vi "Module Top Level.vi"(8 "error in":errorcluster) -> (0 "error out":errorcluster)   [LabVIEW 2018, in "Testing UI 3.lvlib"]
doc: "This is the top level VI for this module. It uses a queue for communications and is stopped user a user event. The general architecture is similar to a simple queued message handler.\n\nThe VIs associated with this module are organized in a LabVIEW Library."
uses:
  Testing UI 3.lvlib
  Private Controls/UI 3 Data.ctl
  Top Level/Shared Controls/APU Setup File.ctl
  Private Controls/Cutoff Frequency.ctl
  Public Controls/Accel Config.ctl
  Private Controls/Module Data.ctl
  Private Controls/Module Action.ctl
  Globals/Host Globals.vi
  Error Handler/Error Handler.lvlib
  File IO/File IO.lvlib
  UDP Writer/PC UDP Writer.lvlib
panel:
  in  "Channel Select":enum16{"Power Section", "Gearbox", "Fan"}(ring)
  in  "Save Accel Config":bool
  in  "Fan Cutoff Frequency":T1={"LP Passband"=1200.0, "HP Stopband"=250.0, "LP Stopband"=1300.0, "HP Passband"=300.0} {"HP Passband" min=1.0 step=1.0 format="%#.4f"; "LP Stopband" min=1.0 step=1.0 format="%#.4f"; "HP Stopband" min=1.0 step=1.0 format="%#.4f"; "LP Passband" min=1.0 step=1.0 format="%#.4f"}
  in  "GB Cutoff Frequency":T1={"LP Passband"=1200.0, "HP Stopband"=250.0, "LP Stopband"=1300.0, "HP Passband"=300.0} {"HP Passband" min=1.0 step=1.0 format="%#.4f"; "LP Stopband" min=1.0 step=1.0 format="%#.4f"; "HP Stopband" min=1.0 step=1.0 format="%#.4f"; "LP Passband" min=1.0 step=1.0 format="%#.4f"}
  in  "PS Cutoff Frequency":T1={"LP Passband"=1200.0, "HP Stopband"=250.0, "LP Stopband"=1300.0, "HP Passband"=300.0} {"HP Passband" min=1.0 step=1.0 format="%#.4f"; "LP Stopband" min=1.0 step=1.0 format="%#.4f"; "HP Stopband" min=1.0 step=1.0 format="%#.4f"; "LP Passband" min=1.0 step=1.0 format="%#.4f"}
  in  "Units Select":string(combo)="0"
  in  "Show Accel?":bool
  out "Accel Cluster":T2
  in  "FAN Sens":dbl=0.0001 caption="Sensitivity (mV/ms-2)" min=0.0001 format="%#.4f"
  in  "GB Sens":dbl=0.0001 caption="Sensitivity (mV/ms-2)" min=0.0001 format="%#.4f"
  in  "PS Sens":dbl=0.0001 caption="Sensitivity (mV/ms-2)" min=0.0001 format="%#.4f"
  out "UI 3 Data":T3
  out "Fan Peak":dbl caption="Velocity PEAK" format="%.2f"
  out "GB RMS":dbl caption="Velocity RMS" format="%.2f"
  out "PS RMS":dbl caption="Velocity RMS" format="%.2f"
  out "Fan RMS Level":dbl(graph)=0.00041195687684329 caption="peaks"
  out "Gearbox RMS Level":dbl(graph)=0.0759733513075506 caption="peaks"
  out "Power Section RMS Level":dbl(graph)=0.022015968164997 caption="peaks"
  out "Fan Peak":dbl(graph)=0.00138609479700936 caption="peaks"
  out "Gearbox Peak":dbl(graph)=0.40103459883114 caption="peaks"
  out "Power Section Peak":dbl(graph)=0.0689049138645727 caption="peaks"
  out "STOP":bool
  # "Vibration Analysis"
  # "Highpass Cutoff Frequency"
  # "Lowpass Cutoff Frequency"
  # "Highpass Cutoff Frequency"
  # "Lowpass Cutoff Frequency"
  # "Highpass Cutoff Frequency"
  # "Lowpass Cutoff Frequency"
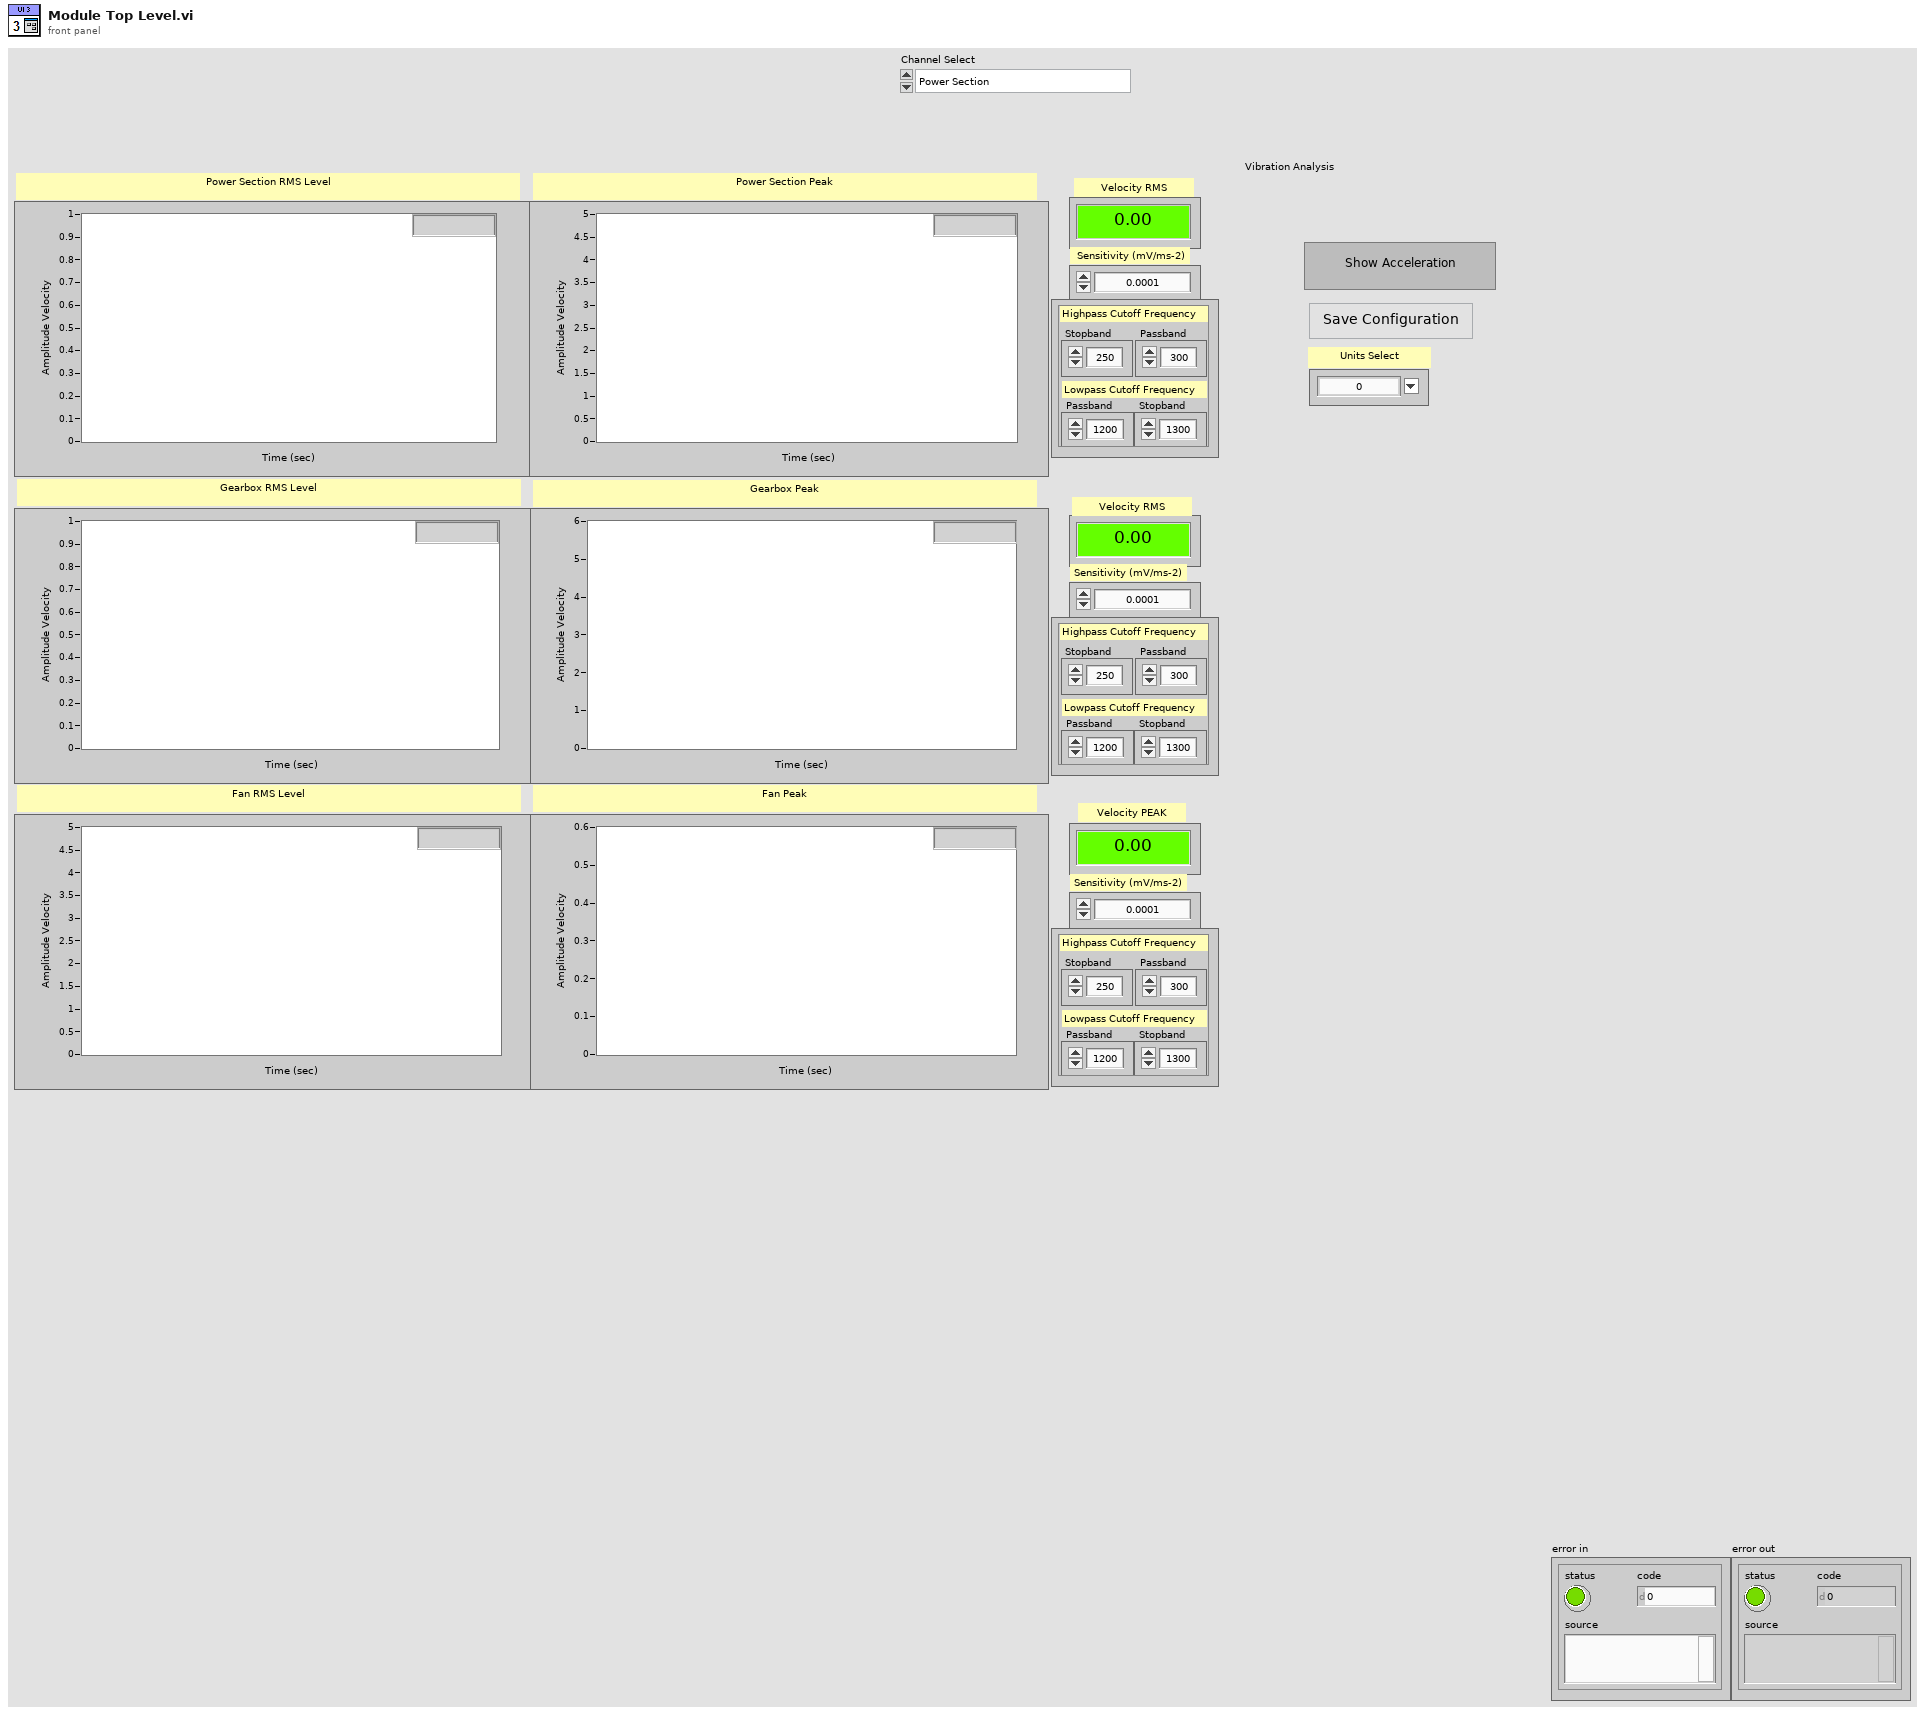
[diagram p1: front panel]
types:
  T1 = typedef "Testing UI 3.lvlib/Cutoff Frequency.ctl" = cluster{"LP Passband":dbl, "HP Stopband":dbl, "LP Stopband":dbl, "HP Passband":dbl}
  T2 = cluster{"Power Section Accel RMS":dbl, "Power Section Accel Peak":dbl, "Gearbox Accel RMS":dbl, "Gearbox Accel Peak":dbl, "Fan Accel RMS":dbl, "Fan Accel Peak":dbl}
  T3 = typedef "Testing UI 3.lvlib/UI 3 Data.ctl" = cluster{"APU Setup File":T4}
  T4 = typedef "APU Setup File.ctl" = cluster{"Sensor Info":string[][], "Variables":string[][], "CMM Table 106":string[][], "CMM Table 106B ":string[][], "Accel Config":string[][], "Report Sheet 1":string[][], "Report Sheet 2":string[][], "Report Sheet 3":string[][]}
  T5 = typedef "Testing UI 3.lvlib/Accel Config.ctl" = cluster{"PS Sens":dbl, "GB Sens":dbl, "FAN Sens":dbl, "PS Cutoff Frequency":T1, "GB Cutoff Frequency":T1, "Fan Cutoff Frequency":T1}
  T6 = enum32{"Invalid", "Standard", "Closed", "Hidden", "Minimized", "Maximized"}
  T7 = typedef "Testing UI 3.lvlib/Module Data.ctl" = cluster{"Data":variant, "Action":T8}
  T8 = typedef "Testing UI 3.lvlib/Module Action.ctl" = enum8{"Init", "Open FP", "Timeout", "Error", "Exit", "Load APU Setup"}
  T9 = typedef "All Data Cluster.ctl" = cluster{"AI":T10, "Accel Data":cluster{"Accel RMS(in/sec2)":dbl[], "Accel Peak(in/sec2)":dbl[], "Velocity RMS(in/sec)":dbl[], "Velocity Peak(in/sec)":dbl[]}, "Temps":cluster{"01-00-9213":dbl[], "01-01-9213":dbl[], "01-02-9213":dbl[]}, "00-03-9402(RPM)":dbl[], "02-04-9871":dbl[], "ARINC":sgl[]}
  T10 = typedef "Acq Data.ctl" = cluster{"00-00-9220":dbl[], "00-01-9220":dbl[], "02-02-9219":dbl[], "02-03-9227":dbl[], "02-05-9205":dbl[]}
  T11 = cluster{"Accel RMS(in/sec2)":dbl[], "Accel Peak(in/sec2)":dbl[], "Velocity RMS(in/sec)":dbl[], "Velocity Peak(in/sec)":dbl[]}
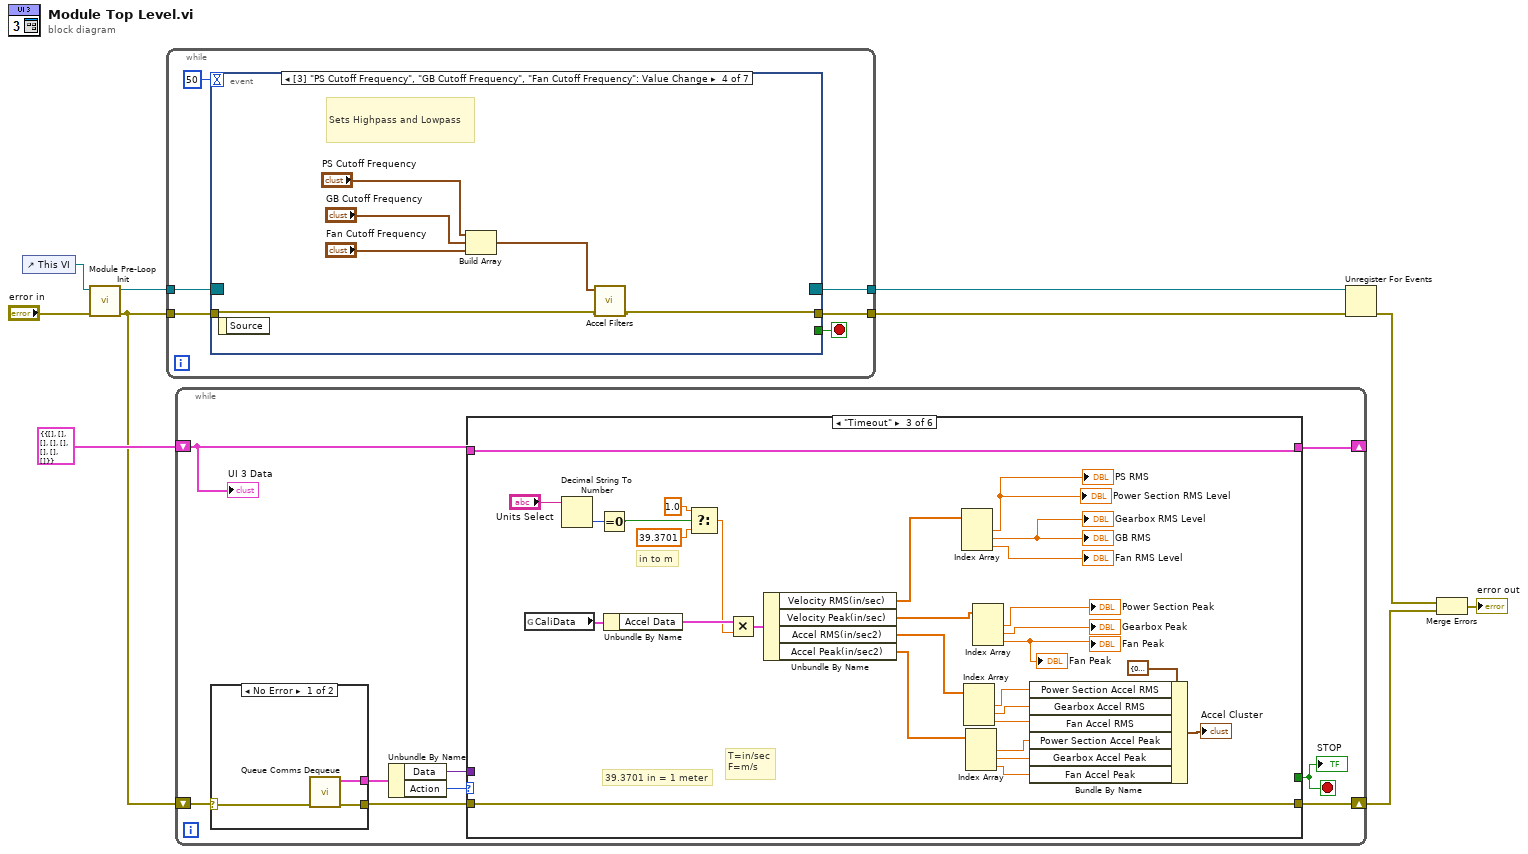
[diagram p0: block diagram]
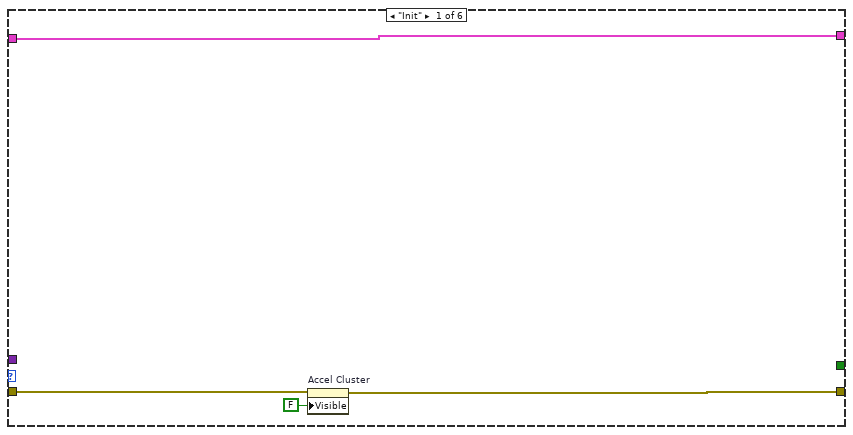
[diagram p2: hidden frame]
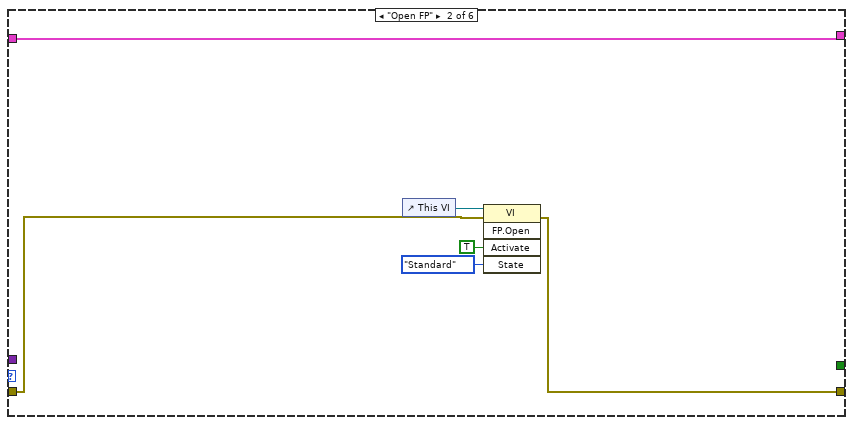
[diagram p3: hidden frame]
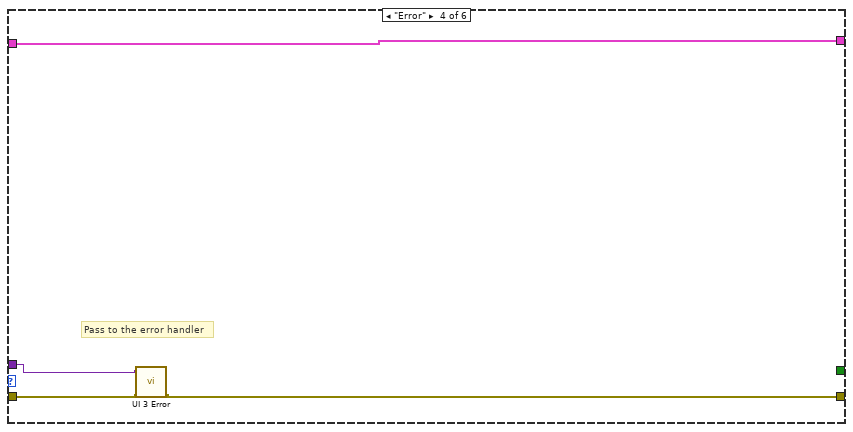
[diagram p4: hidden frame]
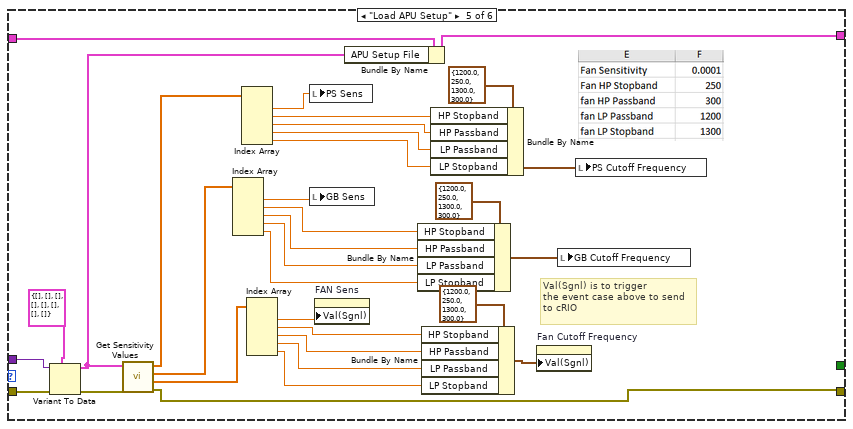
[diagram p5: hidden frame]
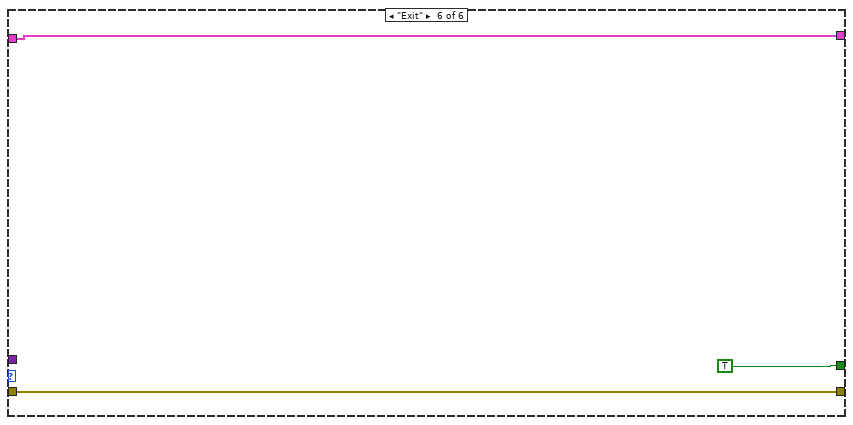
[diagram p6: hidden frame]
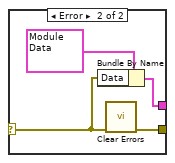
[diagram p7: hidden frame]
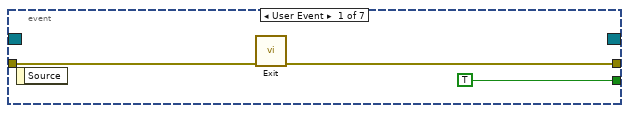
[diagram p8: hidden frame]
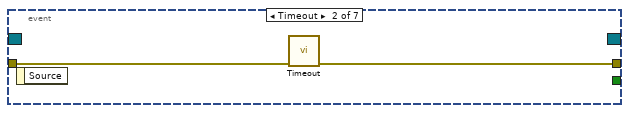
[diagram p9: hidden frame]
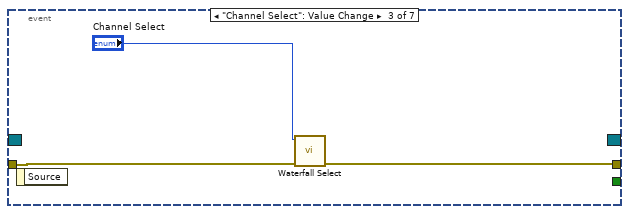
[diagram p10: hidden frame]
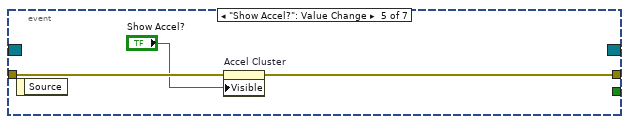
[diagram p11: hidden frame]
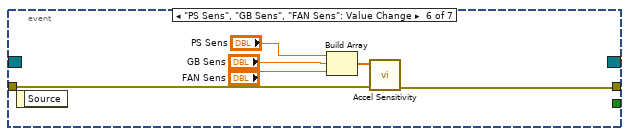
[diagram p12: hidden frame]
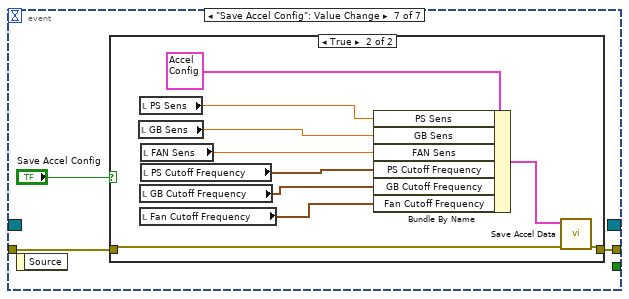
[diagram p13: hidden frame]
diagram:
  n1 = control-ref of="This VI"() -> (w10:refnum<vi>)
  n2 = call "Module Pre-Loop Init.vi"("error in (no error)"="error in", "Top Level VI Ref in"=w10) -> ("error out"=w1:errorcluster, "User Event Stop Ref"=w9:refnum<event-registration>)  [unwired: 8 in]
  n3 = while {
    tunnel: w9 -> [w16]
    tunnel: [w15] -> w7
    tunnel: w1 -> [w14]
    tunnel: [w12] -> w8
    stop <- w13 stop-if-true
    n4 = event shown="[3] \"PS Cutoff Frequency\", \"GB Cutoff Frequency\", \"Fan Cutoff Frequency\": Value Change" {
      selector: w16 -> [_ _ _ _ _ _ _]
      dyn-events: [_ _ _ _ _ _ _] -> w12
      timeout: 50 -> [_ _ _ _ _ _ _]
      tunnel: [w17 w20 w22 w25 w31 w34 w40] -> w15
      tunnel: w14 -> [w18 w21 w24 w26 w33 w35 w42]
      tunnel: [TRUE _ _ _ _ _ _] -> w13
      event User Event {
        n5 = event-data() -> ()  [unwired: 1 in, 1 out]
        n6 = call "Exit.vi"("error in"=w18) -> ("error out"=w17:errorcluster)  [unwired: 10 in]
      }
      event Timeout {
        n7 = event-data() -> ()  [unwired: 1 in, 1 out]
        n8 = call "Timeout.vi"("error in (no error)"=w21) -> ("error out"=w20:errorcluster)  [unwired: 10 in]
      }
      event "Channel Select": Value Change {
        n9 = event-data() -> ()  [unwired: 1 in, 1 out]
        n10 = call "Waterfall Select.vi"("error in (no error)"=w24, "WaterFall Select (0-4)"="Channel Select") -> ("error out"=w22:errorcluster)  [unwired: 9 in]
      }
      event Value Change {
        # "Sets Highpass and Lowpass"
        n11 = event-data() -> ()  [unwired: 1 in, 1 out]
        n12 = Build Array("PS Cutoff Frequency", "GB Cutoff Frequency", "Fan Cutoff Frequency") -> (w27:T1[])
        n13 = call "Accel Filters.vi"("error in (no error)"=w26, "Filters"=w27) -> ("error out"=w25:errorcluster)  [unwired: 9 in]
      }
      event "Show Accel?": Value Change {
        n14 = event-data() -> ()  [unwired: 1 in, 1 out]
        n15 = property on="Accel Cluster" class="Clust (strict)"(error in=w33, "Visible"="Show Accel?") -> (error out=w31:errorcluster)  [unwired: 1 in, 1 out]
      }
      event "PS Sens", "GB Sens", "FAN Sens": Value Change {
        n16 = event-data() -> ()  [unwired: 1 in, 1 out]
        n17 = Build Array("PS Sens", "GB Sens", "FAN Sens") -> (w36:dbl[])
        n18 = call "Accel Sensitivity.vi"("error in (no error)"=w35, "Accel Sensitivities"=w36) -> ("error out"=w34:errorcluster)  [unwired: 9 in]
      }
      event "Save Accel Config": Value Change {
        n19 = event-data() -> ()  [unwired: 1 in, 1 out]
        n20 = case shown="True" "Save Accel Config" {
          tunnel: w42 -> [w43 w53]
          tunnel: [w43 w52] -> w40
          frame False {
          }
          frame True {
            n21 = local read "GB Sens"() -> (w49:dbl)
            n22 = local read "PS Sens"() -> (w50:dbl)
            n23 = local read "GB Cutoff Frequency"() -> (w46:T1)
            n24 = local read "Fan Cutoff Frequency"() -> (w45:T1)
            n25 = local read "FAN Sens"() -> (w48:dbl)
            n26 = local read "PS Cutoff Frequency"() -> (w47:T1)
            n27 = Bundle By Name(cluster=T5 {"PS Sens"=0.0001, "GB Sens"=0.0001, "FAN Sens"=0.0001, "PS Cutoff Frequency"={"LP Passband"=1200.0, "HP Stopband"=250.0, "LP Stopband"=1300.0, "HP Passband"=300.0}, "GB Cutoff Frequency"={"LP Passband"=1200.0, "HP Stopband"=250.0, "LP Stopband"=1300.0, "HP Passband"=300.0}, "Fan Cutoff Frequency"={"LP Passband"=1200.0, "HP Stopband"=250.0, "LP Stopband"=1300.0, "HP Passband"=300.0}}, "PS Sens"=w50, "GB Sens"=w49, "FAN Sens"=w48, "PS Cutoff Frequency"=w47, "GB Cutoff Frequency"=w46, "Fan Cutoff Frequency"=w45) -> (w44:T5)
            n28 = call "Save Accel Data.vi"("error in (no error)"=w53, "Accel Config"=w44) -> ("error out"=w52:errorcluster)  [unwired: 9 in]
          }
        }
      }
    }
  }
  n29 = while {
    shift-right: [w58] -> w6
    shift-left: w1 -> [w57]
    shift-right: [w55] -> _
    shift-left: T3 {"APU Setup File"={"Sensor Info"=[], "Variables"=[], "CMM Table 106"=[], "CMM Table 106B "=[], "Accel Config"=[], "Report Sheet 1"=[], "Report Sheet 2"=[], "Report Sheet 3"=[]}} -> [w56]
    stop <- w54 stop-if-true
    n30 = case shown="No Error" w57 {
      selector: w57 -> [w142 w145]
      tunnel: [w143 w146] -> w62
      tunnel: [w141 w144] -> w59
      frame No Error {
        n31 = call "Queue Comms Dequeue.vi"("error in (no error)"=w142) -> ("error out"=w141:errorcluster, "element"=w143:T7)  [unwired: 9 in]
      }
      frame Error {
        n32 = Bundle By Name(cluster=T7 {"Data"=variant, "Action"=enum."Error"} ("element"), "Data"=w145) -> (w146:T7)
        n33 = call <vilib>:"Clear Errors.vi"("error in (no error)"=w145) -> ("error out"=w144:errorcluster)  [unwired: 5 in, 1 out]
      }
    }
    n34 = Unbundle By Name(w62) -> ("Data"=w60:variant, "Action"=w61:T8)
    n35 = case shown="\"Timeout\"" w61 {
      tunnel: w60 -> [_ _ _ w104 w135 _]
      tunnel: w59 -> [w63 w68 w101 w103 w136 w138]
      tunnel: [w64 w67 w101 w102 w106 w138] -> w58
      tunnel: [_ _ _ _ _ TRUE] -> w54
      tunnel: w56 -> [w66 w72 w100 w105 w137 w139]
      tunnel: [w66 w72 w100 w105 w134 w139] -> w55
      frame "Init" {
        n36 = property on="Accel Cluster" class="Clust (strict)"(error in=w63, "Visible"=FALSE) -> (error out=w64:errorcluster)  [unwired: 1 in, 1 out]
      }
      frame "Open FP" {
        n37 = control-ref of="This VI"() -> (w71:refnum<vi>)
        n38 = invoke class="VI" method="FP.Open"(reference=w71, error in=w68, "Activate"=TRUE ("Activate?"), "State"=T6."Standard") -> (error out=w67:errorcluster)  [unwired: 1 in, 4 out]
      }
      frame "Timeout" {
        # "in to m"
        # "T=in/sec\nF=m/s"
        # "39.3701 in = 1 meter"
        n39 = global read "Host Globals.vi" "CaliData"() -> (w77:T9)
        n40 = Decimal String To Number(string="Units Select") -> (number=w84:i32)  [unwired: 2 in, 1 out]
        n41 = Equal To 0?(x=w84) -> (x = 0?=w85:bool)
        n42 = Unbundle By Name(w77) -> ("Accel Data"=w76:T11)
        n43 = Select(t=1.0, s=w85, f=39.3701) -> (s? t:f=w75:dbl)
        n44 = Multiply(x=w76, y=w75) -> (x*y=w74:T11)
        n45 = Unbundle By Name(w74) -> ("Velocity RMS(in/sec)"=w94:dbl[], "Velocity Peak(in/sec)"=w98:dbl[], "Accel RMS(in/sec2)"=w99:dbl[], "Accel Peak(in/sec2)"=w90:dbl[])
        n46 = Index Array(array=w94) -> (element #1=→"Power Section RMS Level" →"PS RMS":dbl, element #2=→"Gearbox RMS Level" →"GB RMS":dbl, element #3=→"Fan RMS Level":dbl)  [unwired: 3 in]
        n47 = Index Array(array=w99) -> (element #1=w87:dbl, element #2=w88:dbl, element #3=w89:dbl)  [unwired: 3 in]
        n48 = Index Array(array=w90) -> (element #1=w91:dbl, element #2=w92:dbl, element #3=w93:dbl)  [unwired: 3 in]
        n49 = Index Array(array=w98) -> (element #1=→"Power Section Peak":dbl, element #2=→"Gearbox Peak":dbl, element #3=→"Fan Peak" →"Fan Peak":dbl)  [unwired: 3 in]
        n50 = Bundle By Name(cluster=T2 {"Power Section Accel RMS"=0.0, "Power Section Accel Peak"=0.0, "Gearbox Accel RMS"=0.0, "Gearbox Accel Peak"=0.0, "Fan Accel RMS"=0.0, "Fan Accel Peak"=0.0} ("Accel Cluster"), "Power Section Accel RMS"=w87, "Gearbox Accel RMS"=w88, "Fan Accel RMS"=w89, "Power Section Accel Peak"=w91, "Gearbox Accel Peak"=w92, "Fan Accel Peak"=w93) -> (→"Accel Cluster":T2)
      }
      frame "Error" {
        # "Pass to the error handler"
        n51 = call "UI 3 Error.vi"("error in (no error)"=w103, "Data"=w104) -> ("error out"=w102:errorcluster)  [unwired: 9 in]
      }
      frame "Load APU Setup" {
        # "Val(Sgnl) is to trigger\nthe event case above to send\nto cRIO"
        n52 = Variant To Data(error in=w136, type=T4 {"Sensor Info"=[], "Variables"=[], "CMM Table 106"=[], "CMM Table 106B "=[], "Accel Config"=[], "Report Sheet 1"=[], "Report Sheet 2"=[], "Report Sheet 3"=[]} ("APU Setup File"), Variant=w135) -> (data=w131:T4, error out=w132:errorcluster)
        n53 = call "Get Sensitivity Values.vi"("error in (no error)"=w132, "APU Setup File"=w131) -> ("Error Out"=w106:errorcluster, "Fan"=w126:dbl[], "GS"=w128:dbl[], "PS"=w130:dbl[])  [unwired: 6 in]
        n54 = Index Array(array=w128) -> (element #1=w127:dbl, element #2=w116:dbl, element #3=w115:dbl, element #4=w114:dbl, element #5=w113:dbl)  [unwired: 5 in]
        n55 = Index Array(array=w130) -> (element #1=w129:dbl, element #2=w122:dbl, element #3=w121:dbl, element #4=w120:dbl, element #5=w119:dbl)  [unwired: 5 in]
        n56 = Index Array(array=w126) -> (element #1=w125:dbl, element #2=w111:dbl, element #3=w110:dbl, element #4=w109:dbl, element #5=w108:dbl)  [unwired: 5 in]
        n57 = local write "PS Sens"(w129) -> ()
        n58 = local write "GB Sens"(w127) -> ()
        n59 = property on="FAN Sens" class="DigNum (strict)"("Val(Sgnl)"=w125) -> ()  [unwired: 2 in, 2 out]
        n60 = Bundle By Name(cluster=w137, "APU Setup File"=w131) -> (w134:T3)
        n61 = Bundle By Name(cluster=T1 {"LP Passband"=1200.0, "HP Stopband"=250.0, "LP Stopband"=1300.0, "HP Passband"=300.0} ("PS Cutoff Frequency"), "HP Stopband"=w116, "HP Passband"=w115, "LP Passband"=w114, "LP Stopband"=w113) -> (w117:T1)
        n62 = Bundle By Name(cluster=T1 {"LP Passband"=1200.0, "HP Stopband"=250.0, "LP Stopband"=1300.0, "HP Passband"=300.0} ("PS Cutoff Frequency"), "HP Stopband"=w111, "HP Passband"=w110, "LP Passband"=w109, "LP Stopband"=w108) -> (w107:T1)
        n63 = Bundle By Name(cluster=T1 {"LP Passband"=1200.0, "HP Stopband"=250.0, "LP Stopband"=1300.0, "HP Passband"=300.0} ("PS Cutoff Frequency"), "HP Stopband"=w122, "HP Passband"=w121, "LP Passband"=w120, "LP Stopband"=w119) -> (w123:T1)
        n64 = property on="Fan Cutoff Frequency" class="Clust (strict)"("Val(Sgnl)"=w107) -> ()  [unwired: 2 in, 2 out]
        n65 = local write "GB Cutoff Frequency"(w117) -> ()
        n66 = local write "PS Cutoff Frequency"(w123) -> ()
      }
      frame "Exit" {
      }
    }
    "STOP" <- w54
    "UI 3 Data" <- w56
  }
  n67 = Unregister For Events(event registration refnum=w8, error in=w7) -> (error out=w4:errorcluster)
  n68 = Merge Errors(w4, w6) -> (→"error out":errorcluster)
